vi "Write Adaptive FF IIR coeffs.vi"(9 "Fs [MHz}":dbl min=0.0 max=1.0, 10 "cutoff fequency [MHz]":dbl min=0.0 max=10000.0, 11 "FpgaRef5785 in":refnum<class "FpgaRef5782.lvclass">) -> (3 "FpgaRef5785 out":refnum<class "FpgaRef5782.lvclass">)   [LabVIEW 2018]
uses:
  FpgaRef/FpgaRef5782/FpgaRef5782.lvclass
  C:/PXIe/InProgress/source/Host/FpgaRef/FpgaRefBase/FpgaRefBase.lvclass
  FPGA/fpga_settings.ctl
  <vilib>/rvi/FXPMathLib/FxpInterpret/XNode/nifxpmath_Interpret.xnode
  FpgaRef/FpgaRefBase/FpgaRefBase.lvclass
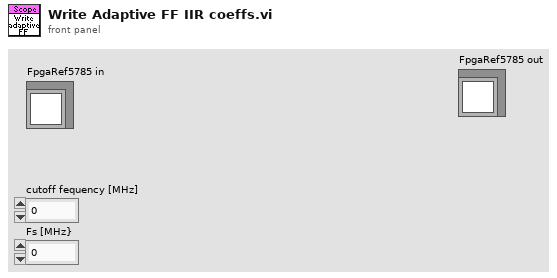
[diagram p1: front panel]
types:
  T1 = typedef "fpga_settings.ctl" = enum16{"Feedback Enable", "New FIR coeffs", "FIR shift", "Enable filter", "Set Downsample", "Downsample", "CIC Gain", "Record length", "Trigger samples", "Quiet time", "a_am", "b_am", "Use fixed delay", "fixed sin_fi", "fixed cos_fi", "Ki*Tau", "Kp", "Kd_Tau", "Fi_start", "Fi_delta", "DC_offs 0", "DC_offs 1", "DC_offs 2", "DC_offs 3", "Ki*Tau am", "Kp am", "Kd_Tau am", "Feedback AM", "Trigger delay", "Feedback delay", "Setpoint enable", "Beam enable", "Samples to acquire", "Cavity Enable", "Cavity C1", "Cavity C2", "Cavity C3", "Cavity C4", "Cavity C5", "Input delay", "Ki*Tau Q", "Kp Q", "Kd_Tau Q", "Adaptive FF enable", "Feedforward a0", "Feedforward b0", "FF src adress", "FF dest adress", "Output scale", "Input scale", "Host scale", "FF_IIR b0", "FF_IIR b1", "FF_IIR b2", "FF_IIR-a1", "FF_IIR-a2", "Enable HW trigger"}
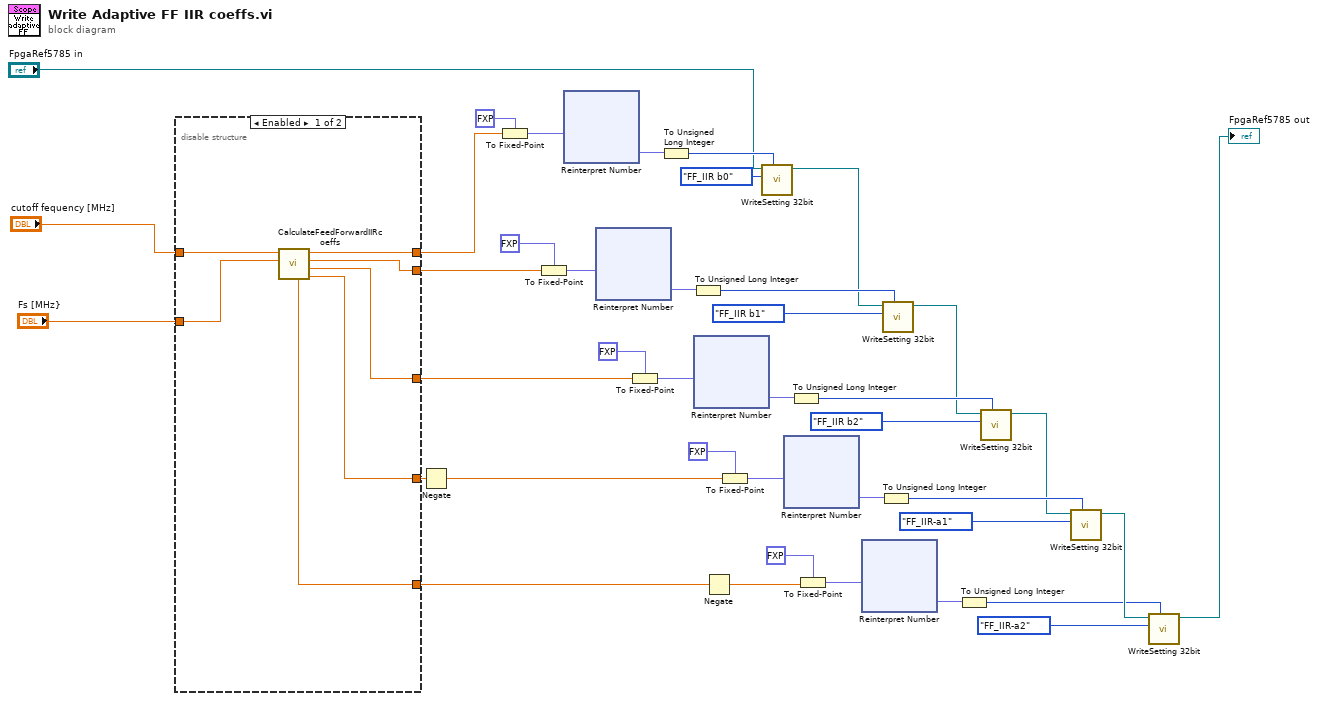
[diagram p0: block diagram]
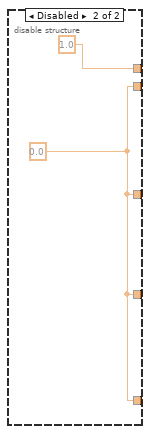
[diagram p2: hidden frame]
diagram:
  n1 = disable-structure shown="Enabled" {
    disable-tunnel: "cutoff fequency [MHz]" -> [w47 _]
    disable-tunnel: "Fs [MHz}" -> [w46 _]
    disable-tunnel: [w45 1.0] -> w28
    disable-tunnel: [w44 w49] -> w26
    disable-tunnel: [w43 w49] -> w7
    disable-tunnel: [w42 w49] -> w6
    disable-tunnel: [w41 w49] -> w4
    frame Enabled {
      n2 = call "CalculateFeedForwardIIRcoeffs.vi"("fs [MHz]"=w46, "fc [MHz]"=w47) -> ("a1"=w42:dbl, "b2"=w43:dbl, "b1"=w44:dbl, "b0"=w45:dbl, "a2"=w41:dbl)  [unwired: 5 in]
    }
    frame Disabled {
      w49 = 0.0
    }
  }
  n3 = Negate(x=w6) -> (-x=w5:dbl)
  n4 = To Fixed-Point(fixed-point type=fxp<+/-,32,2> 0.0 ("x"), number=w28) -> (fixed-point=w39:fxp<+/-,32,2>)
  n5 = To Fixed-Point(fixed-point type=fxp<+/-,32,2> 0.0 ("x"), number=w26) -> (fixed-point=w33:fxp<+/-,32,2>)
  n6 = xnode "Reinterpret Number"("x"=w39) -> ("y"=w40:fxp<+,32,32>)
  n7 = xnode "Reinterpret Number"("x"=w33) -> ("y"=w32:fxp<+,32,32>)
  n8 = To Fixed-Point(fixed-point type=fxp<+/-,32,2> 0.0 ("x"), number=w7) -> (fixed-point=w23:fxp<+/-,32,2>)
  n9 = To Unsigned Long Integer(number=w40) -> (unsigned 32bit integer=w38:u32)
  n10 = To Unsigned Long Integer(number=w32) -> (unsigned 32bit integer=w35:u32)
  n11 = xnode "Reinterpret Number"("x"=w23) -> ("y"=w24:fxp<+,32,32>)
  n12 = Negate(x=w4) -> (-x=w1:dbl)
  n13 = To Fixed-Point(fixed-point type=fxp<+/-,32,2> 0.0 ("x"), number=w5) -> (fixed-point=w16:fxp<+/-,32,2>)
  n14 = call "WriteSetting 32bit.vi"("value"=w38, "FPGA Setting"=fpga_settings."FF_IIR b0", "FpgaRefBase in"="FpgaRef5785 in") -> ("FpgaRefBase out"=w31:refnum<class "FpgaRef5782.lvclass">)  [unwired: 7 in, 1 out]
  n15 = xnode "Reinterpret Number"("x"=w16) -> ("y"=w15:fxp<+,32,32>)
  n16 = To Unsigned Long Integer(number=w24) -> (unsigned 32bit integer=w21:u32)
  n17 = To Fixed-Point(fixed-point type=fxp<+/-,32,2> 0.0 ("x"), number=w1) -> (fixed-point=w2:fxp<+/-,32,2>)
  n18 = xnode "Reinterpret Number"("x"=w2) -> ("y"=w14:fxp<+,32,32>)
  n19 = To Unsigned Long Integer(number=w15) -> (unsigned 32bit integer=w18:u32)
  n20 = call "WriteSetting 32bit.vi"("value"=w35, "FPGA Setting"=fpga_settings."FF_IIR b1", "FpgaRefBase in"=w31) -> ("FpgaRefBase out"=w11:refnum<class "FpgaRef5782.lvclass">)  [unwired: 7 in, 1 out]
  n21 = To Unsigned Long Integer(number=w14) -> (unsigned 32bit integer=w3:u32)
  n22 = call "WriteSetting 32bit.vi"("value"=w21, "FPGA Setting"=fpga_settings."FF_IIR b2", "FpgaRefBase in"=w11) -> ("FpgaRefBase out"=w10:refnum<class "FpgaRef5782.lvclass">)  [unwired: 7 in, 1 out]
  n23 = call "WriteSetting 32bit.vi"("value"=w18, "FPGA Setting"=fpga_settings."FF_IIR-a1", "FpgaRefBase in"=w10) -> ("FpgaRefBase out"=w9:refnum<class "FpgaRef5782.lvclass">)  [unwired: 7 in, 1 out]
  n24 = call "WriteSetting 32bit.vi"("value"=w3, "FPGA Setting"=fpga_settings."FF_IIR-a2", "FpgaRefBase in"=w9) -> ("FpgaRefBase out"=→"FpgaRef5785 out":refnum<class "FpgaRef5782.lvclass">)  [unwired: 7 in, 1 out]
